vi "SetHidden.vi"(8 "error in (no error)":errorcluster, 10 "Hidden?":bool, 11 "FolloWin in":refnum<class "FolloWin.lvclass">) -> (0 "error out":errorcluster, 3 "FolloWin out":refnum<class "FolloWin.lvclass">)   [LabVIEW 2023, in "FolloWin.lvclass"]
doc: "Sets FolloWin window to be hidden or not."
uses:
  FolloWin.lvclass
  FolloWin.lvclass/FolloWin.ctl
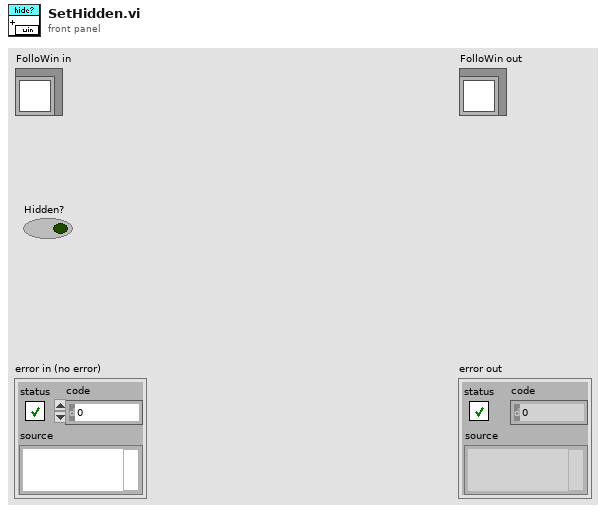
[diagram p1: front panel]
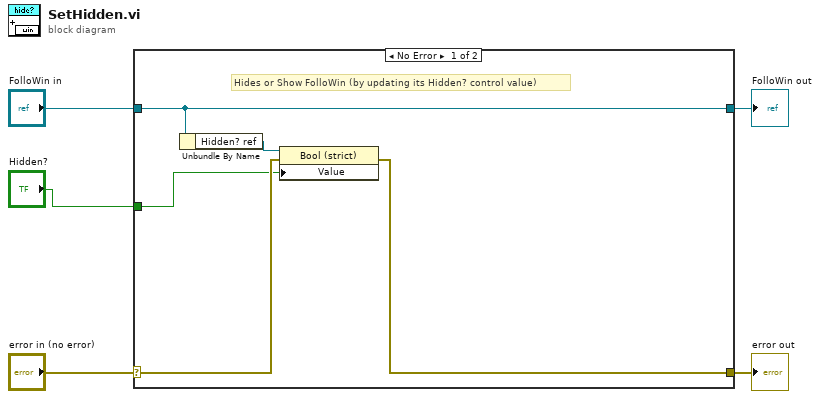
[diagram p0: block diagram]
diagram:
  n1 = case shown="No Error" "error in (no error)" {
    selector: "error in (no error)" -> [w8 w12]
    tunnel: [w7 w12] -> w4
    tunnel: [w10 w11] -> w2
    tunnel: "FolloWin in" -> [w10 w11]
    tunnel: "Hidden?" -> [w6 _]
    frame No Error {
      # "Hides or Show FolloWin (by updating its Hidden? control value)"
      n2 = Unbundle By Name(w10) -> ("Hidden? ref"=w9:refnum<vi>)
      n3 = property on="Property Node" class="Bool (strict)"(reference=w9, error in=w8, "Value"=w6) -> (error out=w7:errorcluster)  [unwired: 1 out]
    }
    frame Error {
    }
  }
  "error out" <- w4
  "FolloWin out" <- w2
